vi "System Explorer - Add extra pages to System Explorer library.vi"(8 "error in (no error)":errorcluster, 10 "CD Wizard - Internal Data":T1, 11 "ProjectItem IN":refnum<vi>) -> (0 "error out":errorcluster, 3 "ProjectItem OUT":refnum<vi>)   [LabVIEW 2015]
doc: "Create an addition folder under the ProjectItem and add all created extra pages to this folder."
uses:
  TypDef/CD Wizard - Internal data.ctl
  TypDef/CD Wizard - Execution Mode.ctl
  TypDef/CD Wizard - Extra Page Name and GUID.ctl
  Constants/Constants TypDef/CD System Explorer lvlib.ctl
  TypDef/Add Item - Type.ctl
  Constants/CD System Explorer lvlib.vi
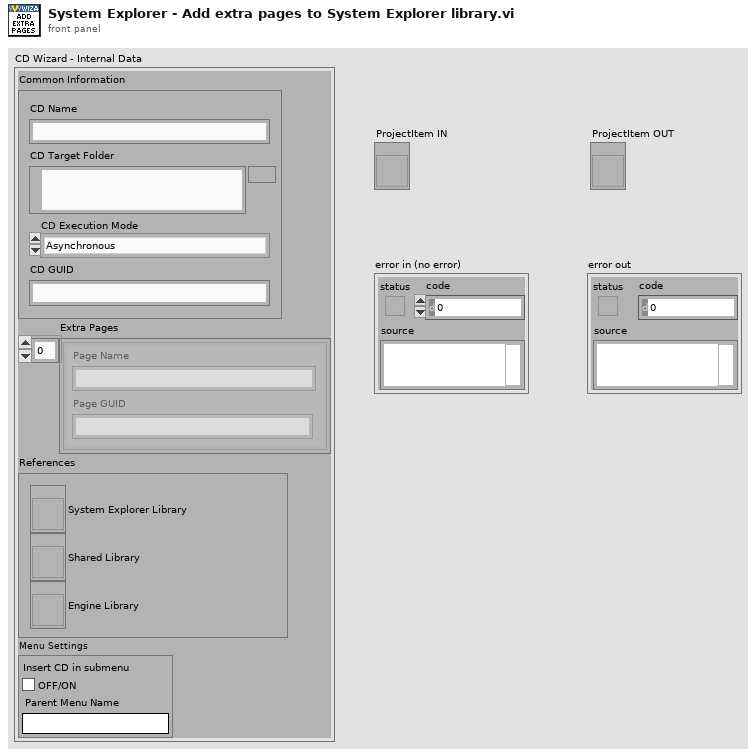
[diagram p1: front panel]
types:
  T1 = typedef "CD Wizard - Internal data.ctl" = cluster{"Common Information":cluster{"CD Name":string, "CD Target Folder":path, "CD Execution Mode":T2, "CD GUID":string}, "Extra Pages":T3[], "References":cluster{"System Explorer Library":refnum<vi>, "Shared Library":refnum<vi>, "Engine Library":refnum<vi>}, "Menu Settings":cluster{"Insert CD in submenu":bool, "Parent Menu Name":string}}
  T2 = typedef "CD Wizard - Execution Mode.ctl" = enum16{"Asynchronous", "Inline HW Interface", "Inline Model Interface", "Inline Timing and Sync", "Asynchronous Timing and Sync"}
  T3 = typedef "CD Wizard - Extra Page Name and GUID.ctl" = cluster{"Page Name":string, "Page GUID":string}
  T4 = typedef "CD System Explorer lvlib.ctl" = enum16{"LibraryFileName", "LibraryFolderName", "System Explorer.FolderName", "System Explorer.Dynamically Called.FolderName", "System Explorer.Dynamically Called.Extra Pages.FolderName", "System Explorer.Dynamically Called.Extra Pages.TemplatePathAndName", "System Explorer.Dynamically Called.Main Page.VIName", "System Explorer.Dynamically Called.Main Page.TemplatePathAndName", "System Explorer.Dynamically Called.Initialization VI.VIName", "System Explorer.Dynamically Called.Initialization VI.TemplatePathAndName", "System Explorer.SubVI.FolderName", "System Explorer.Types.FolderName"}
  T5 = typedef "Add Item - Type.ctl" = string
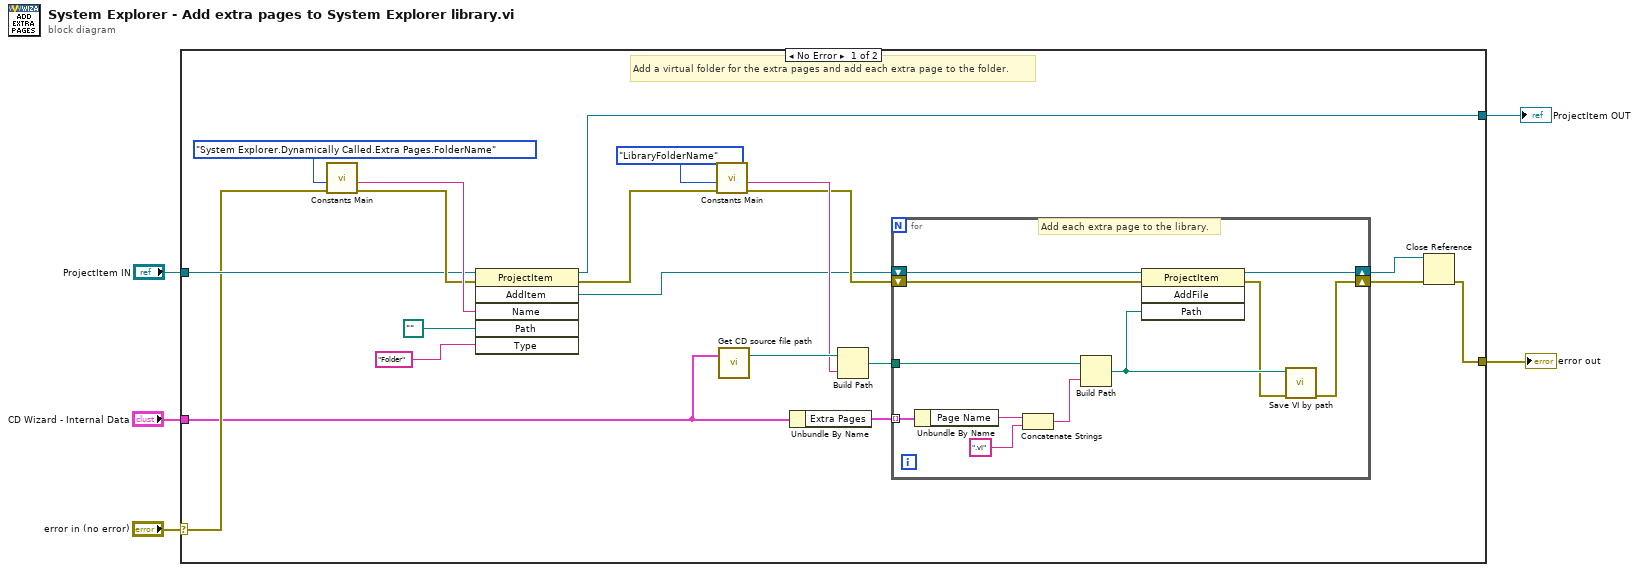
[diagram p0: block diagram]
diagram:
  n1 = case shown="No Error" "error in (no error)" {
    selector: "error in (no error)" -> [w19 w38]
    tunnel: [w7 w38] -> w4
    tunnel: "CD Wizard - Internal Data" -> [w12 _]
    tunnel: "ProjectItem IN" -> [w20 w37]
    tunnel: [w9 w37] -> w1
    frame No Error {
      # "Add a virtual folder for the extra pages and add each extra page to the folder."
      n2 = call-poly "Constants Main.vi"("error in (no error)"=w19, "Action"=CD_System_Explorer_lvlib."System Explorer.Dynamically Called.Extra Pages.FolderName") -> ("error out"=w22:errorcluster, "Output"=w23:string)  [unwired: 8 in]
      n3 = invoke class="ProjectItem" method="AddItem"(reference=w20, error in=w22, "Name"=w23, "Path"=path "", "Type"=T5 "Folder" ("Add Item - Type")) -> (reference out=w9:refnum<vi>, error out=w14:errorcluster, "AddItem"=w10:refnum<vi>)  [unwired: 1 in, 3 out]
      n4 = call-poly "Constants Main.vi"("error in (no error)"=w14, "Action"=CD_System_Explorer_lvlib."LibraryFolderName") -> ("error out"=w13:errorcluster, "Output"=w15:string)  [unwired: 8 in]
      n5 = call "Get CD source file path.vi"("CD Wizard - Internal Data"=w12) -> ("CD Source file path"=w17:path)  [unwired: 2 in]
      n6 = Unbundle By Name(w12) -> ("Extra Pages"=w18:T3[])
      n7 = Build Path(base path=w17, name or relative path=w15) -> (appended path=w11:path)
      n8 = for {
        tunnel: w18 -> [w31] mode=indexing
        shift-right: [w34] -> w6
        shift-left: w10 -> [w36]
        shift-right: [w26] -> w8
        shift-left: w13 -> [w35]
        tunnel: w11 -> [w29]
        # "Add each extra page to the library."
        n9 = Unbundle By Name(w31) -> ("Page Name"=w32:string)
        n10 = Concatenate Strings(w32, ".vi") -> (w30:string)
        n11 = Build Path(base path=w29, name or relative path=w30) -> (appended path=w28:path)
        n12 = invoke class="ProjectItem" method="AddFile"(reference=w36, error in=w35, "Path"=w28) -> (reference out=w34:refnum<vi>, error out=w27:errorcluster)  [unwired: 1 in, 2 out]
        n13 = call "Save VI by path.vi"("error in (no error)"=w27, "VI path"=w28) -> ("error out"=w26:errorcluster)  [unwired: 9 in]
      }
      n14 = Close Reference(reference=w6, error in (no error)=w8) -> (error out=w7:errorcluster)
    }
    frame Error {
      # "Output default values."
    }
  }
  "error out" <- w4
  "ProjectItem OUT" <- w1
